vi "Write Network Slave.vi"(8 "error in":errorcluster, 10 "network slave":refnum<class "Network Slave.lvclass">, 11 "Modbus slave in":refnum<class "Modbus Slave.lvclass">) -> (0 "error out":errorcluster, 3 "Modbus slave out":refnum<class "Modbus Slave.lvclass">)   [LabVIEW 2015, in "Modbus Library.lvlib" / "Modbus Slave.lvclass"]
doc: "This VI is an accessor for the <B>network slave</B> stored in the Modbus slave instance. This accessor can be used as a property node. This network slave is used by the Modbus instance to communicate on the physical bus."
uses:
  Modbus Slave.lvclass
  Network Protocol/Network Slave/Network Slave.lvclass
  Modbus Slave.lvclass/Modbus Slave.ctl
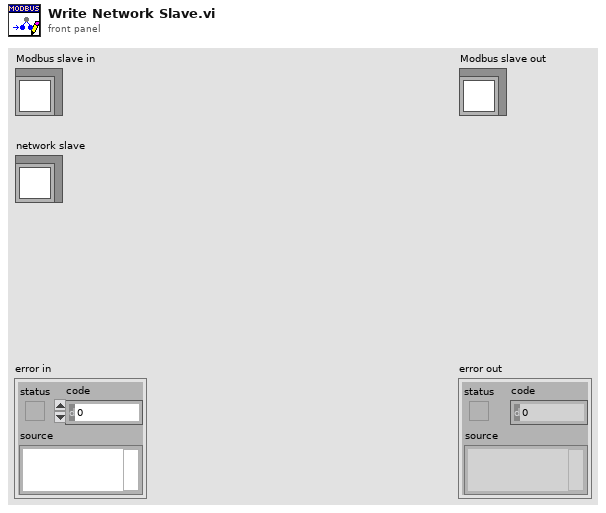
[diagram p1: front panel]
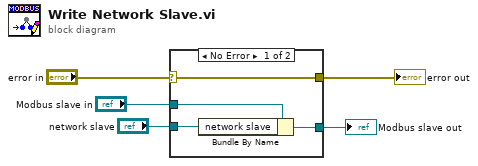
[diagram p0: block diagram]
diagram:
  n1 = case shown="No Error" "error in" {
    selector: "error in" -> [w9 w10]
    tunnel: [w9 w10] -> w4
    tunnel: [w7 w11] -> w2
    tunnel: "Modbus slave in" -> [w8 w11]
    tunnel: "network slave" -> [w6 _]
    frame No Error {
      n2 = Bundle By Name(cluster=w8, "network slave"=w6) -> (w7:refnum<class "Modbus Slave.lvclass">)
    }
    frame Error {
    }
  }
  "error out" <- w4
  "Modbus slave out" <- w2
